vi "merge_Count Up.vi"   [LabVIEW 2017, in "NI_FunctionBlockMergeVIs.lvlib"]
doc: "Counts up from zero. The <B>counter value</B> output increments on each rising edge of the <B>count up</B> input. The <B>done</B> output returns TRUE when <B>counter value</B> is greater than or equal to <B>preset value</B>."
uses:
  <vilib>/functionblocks/NI_FunctionBlockMergeVIs.lvlib
  <vilib>/functionblocks/FB Core/FB Core.xnode
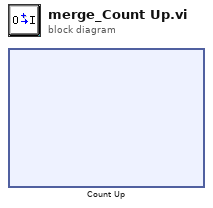
[diagram p0: block diagram]
diagram:
  n1 = xnode "Count Up"() -> ()  [unwired: 4 in, 3 out]
